vi "用户登录.vi"(8 "error in (no error)":errorcluster caption="错误输入（无错误）", 9 "Password":string caption="密   码:", 11 "UserName":string caption="用户名:") -> (0 "error out":errorcluster caption="错误输出", 1 "ErrorMessage":string, 2 "登录成功":bool)   [LabVIEW 2015]
uses:
  mes/ctl/SenduserRightVerify.ctl
  Global.vi
  mes/ctl/ReceiveuserRightVerify.ctl
panel:
  in  "Headers":string[][](array[string])=[["Content-Type", "text/xml;charset=UTF-8"], ["SOAPAction", "\"http://tempuri.org/IUserRightVerifyServiceImpl/UserRightVerify\""], ["Connection", "Keep-Alive"], ["User-Agent", "Apache-HttpClient/4.1.1 (java 1.5)"]]
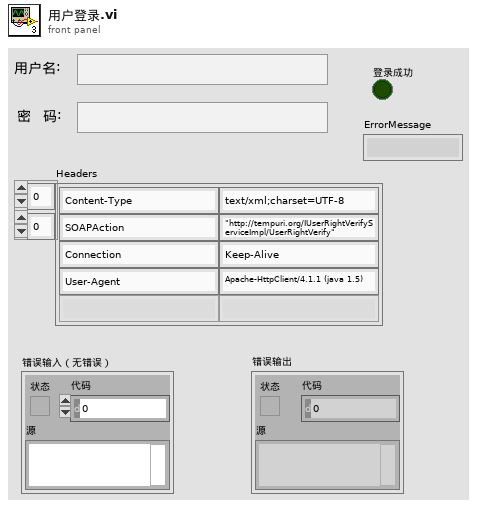
[diagram p1: front panel]
types:
  T1 = typedef "SenduserRightVerify.ctl" = cluster{"#attributes":cluster{"xmlns:soapenv":string, "xmlns:tem":string, "xmlns:cal":string}, "soapenv:Header":string, "soapenv:Body":cluster{"tem:UserRightVerify":cluster{"tem:model":cluster{"cal:equipNum":string, "cal:passWord":string, "cal:siteCode":string, "cal:userName":string}}}}
  T2 = cluster{"接口地址(URL)":string, "权限校验":string, "产品进站":string, "参数采集":string, "产品出站":string, "设备状态":string, "设备编号(equipNum)":string, "站点名称(siteCode)":string, "生产类型(productType)":string, "试验单号(testOrderNum)":string}
  T3 = typedef "ReceiveuserRightVerify.ctl" = cluster{"#attributes":cluster{"xmlns:s":string}, "s:Body":cluster{"UserRightVerifyResponse":cluster{"#attributes":cluster{"xmlns":string}, "UserRightVerifyResult":cluster{"#attributes":cluster{"xmlns:a":string, "xmlns:i":string}, "a:ErrorCode":string, "a:ErrorMessage":string, "a:Success":string}}}}
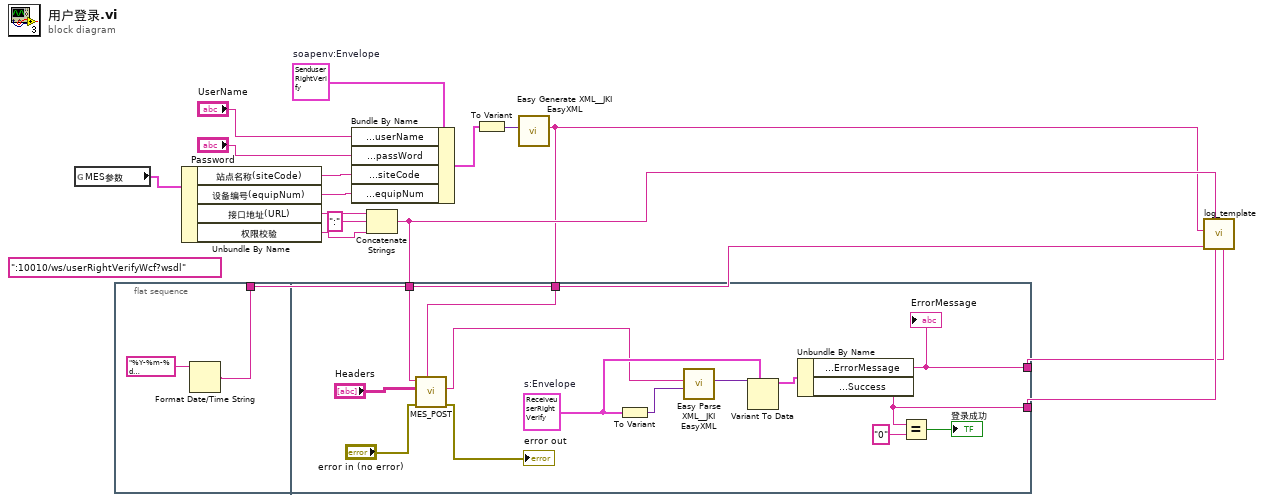
[diagram p0: block diagram]
diagram:
  w8 = T1 {"#attributes"={"xmlns:soapenv"="http://schemas.xmlsoap.org/soap/envelope/", "xmlns:tem"="http://tempuri.org/", "xmlns:cal"="http://schemas.datacontract.org/2004/07/CalbUserRightVerifyService"}, "soapenv:Header"="", "soapenv:Body"={"tem:UserRightVerify"={"tem:model"={"cal:equipNum"="", "cal:passWord"="", "cal:siteCode"="", "cal:userName"=""}}}}  # soapenv:Envelope
  (unwired) ":10010/ws/userRightVerifyWcf?wsdl"
  n1 = global read "Global.vi" "MES参数"() -> (w12:T2)
  n2 = flat-sequence {
    tunnel: [w17] -> w3
    tunnel: w5 -> [w32]
    tunnel: w4 -> [w23]
    tunnel: [w20] -> w2
    tunnel: [w19] -> w1
    frame #0 {
      n3 = Format Date/Time String(time format string (%c)="%Y-%m-%d %H:%M:%S%3u-->" ("EndTime")) -> (date/time string=w17:string)  [unwired: 2 in]
    }
    frame #1 {
      w25 = T3 {"#attributes"={"xmlns:s"="http://schemas.xmlsoap.org/soap/envelope/"}, "s:Body"={"UserRightVerifyResponse"={"#attributes"={"xmlns"="http://tempuri.org/"}, "UserRightVerifyResult"={"#attributes"={"xmlns:a"="http://schemas.datacontract.org/2004/07/EdgeUtility", "xmlns:i"="http://www.w3.org/2001/XMLSchema-instance"}, "a:ErrorCode"="", "a:ErrorMessage"="", "a:Success"=""}}}}  # s:Envelope
      n4 = call "MES_POST.vi"("DATA"=w23, "错误输入（无错误）"="error in (no error)", 10:"Headers", "URL"=w32) -> ("错误输出"=→"error out":errorcluster, "body"=w22:string)  [unwired: 5 in, 1 out]
      n5 = To Variant(anything=w25) -> (Variant=w31:variant)
      n6 = call <vilib>:"Easy Parse XML__JKI EasyXML.vi"("LabVIEW Data (Type)"=w31, "XML String"=w22) -> ("LabVIEW Data"=w30:variant)  [unwired: 8 in, 1 out]
      n7 = Variant To Data(type=w25, Variant=w30) -> (data=w29:T3)  [unwired: 1 in, 1 out]
      n8 = Unbundle By Name(w29) -> ("s:Body.UserRightVerifyResponse.UserRightVerifyResult.a:ErrorMessage"=w19:string, "s:Body.UserRightVerifyResponse.UserRightVerifyResult.a:Success"=w20:string)
      "ErrorMessage" <- w19
      n9 = Equal?(x=w20, y="0") -> (x = y?=→"登录成功":bool)
    }
  }
  n10 = Unbundle By Name(w12) -> ("站点名称(siteCode)"=w13:string, "设备编号(equipNum)"=w14:string, "接口地址(URL)"=w9:string, "权限校验"=w6:string)
  n11 = Bundle By Name(cluster=w8, "soapenv:Body.tem:UserRightVerify.tem:model.cal:userName"="UserName", "soapenv:Body.tem:UserRightVerify.tem:model.cal:passWord"="Password", "soapenv:Body.tem:UserRightVerify.tem:model.cal:siteCode"=w13, "soapenv:Body.tem:UserRightVerify.tem:model.cal:equipNum"=w14) -> (w16:T1)
  n12 = Concatenate Strings(w9, ":" ("字符串"), w6) -> (w5:string)
  n13 = To Variant(anything=w16) -> (Variant=w15:variant)
  n14 = call <vilib>:"Easy Generate XML__JKI EasyXML.vi"("LabVIEW Data"=w15) -> ("XML String"=w4:string)  [unwired: 9 in, 1 out]
  n15 = call "log_template.vi"(4:w1, 6:w2, 7:w5, 8:w3, 10:w4) -> ()  [unwired: 7 in]
